vi "Read Mode.vi"(8 "error in (no error)":errorcluster, 11 "String Compare in":refnum<class "String Compare.lvclass">) -> (0 "error out":errorcluster, 2 "Mode":T1, 3 "String Compare out":refnum<class "String Compare.lvclass">)   [LabVIEW 2015, in "String Compare.lvclass"]
uses:
  String Compare.lvclass
  Config/Mode.ctl
  String Compare.lvclass/String Compare.ctl
  Config/String Compare Config.lvclass
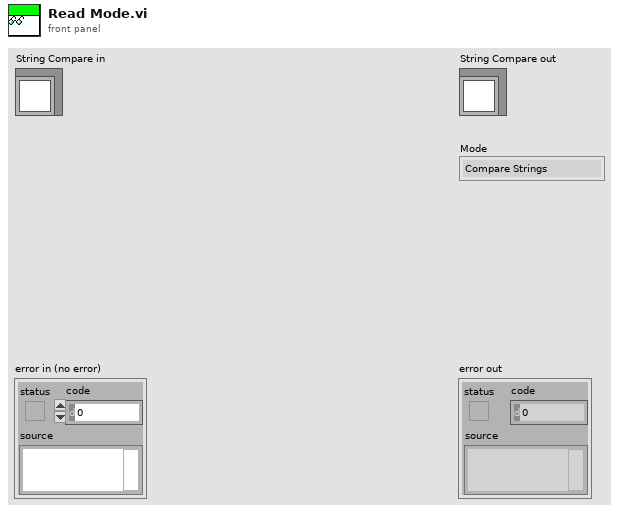
[diagram p1: front panel]
types:
  T1 = typedef "String Compare Config.lvclass/Mode.ctl" = enum16{"Compare Strings", "Match Regex"}
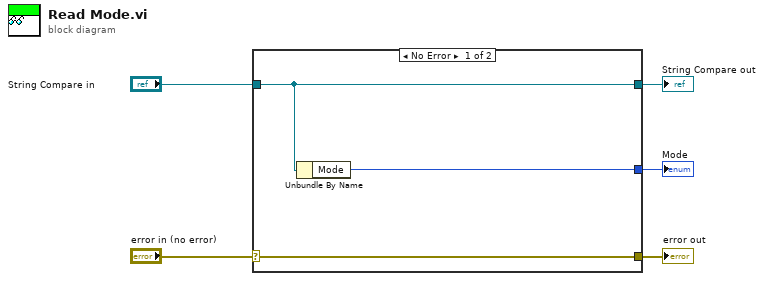
[diagram p0: block diagram]
diagram:
  n1 = case shown="No Error" "error in (no error)" {
    selector: "error in (no error)" -> [w8 w9]
    tunnel: [w8 w9] -> w4
    tunnel: [w7 w10] -> w2
    tunnel: "String Compare in" -> [w7 w10]
    tunnel: [w6 _] -> w1
    frame No Error {
      n2 = Unbundle By Name(w7) -> ("Mode"=w6:T1)
    }
    frame Error {
    }
  }
  "error out" <- w4
  "String Compare out" <- w2
  "Mode" <- w1
